vi "Utility Fast Comms.vi"(8 "Fast Comms":bool, 11 "Command":string) -> (3 "Fast Command":string)   [LabVIEW 2018, in "ChromTech MX-Class Drivers.lvlib"]
doc: "Appends a carriage return to the end of the command, indicating the end of a transmitted string. This will cause the pump to immediately respond to the received command, and may help speed communications."
uses:
  <instrlib>/ChromTech MX-Class Pump/ChromTech MX-Class Drivers.lvlib
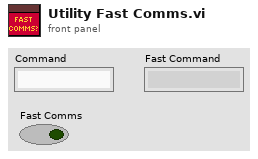
[diagram p1: front panel]
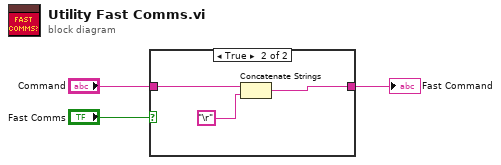
[diagram p0: block diagram]
diagram:
  n1 = case shown="True" "Fast Comms" {
    tunnel: "Command" -> [w4 w7]
    tunnel: [w4 w5] -> w3
    frame False {
    }
    frame True {
      n2 = Concatenate Strings(w7, "\r") -> (w5:string)
    }
  }
  "Fast Command" <- w3
